vi "QR_code_Check_St2.vi"(5 "Columns":string[](array[string]), 8 "error in (no error)":errorcluster, 9 "replace %s":string, 10 "table":string, 11 "Refnum in":T1) -> (0 "error out":errorcluster, 2 "TRUE no barcode Done on station 1":bool, 3 "Refnum out":T1, 4 "FALSE healty":bool, 6 "resulting string":string, 7 "TRUE Duplication on Station 2":bool)   [LabVIEW 2017]
uses:
  <vilib>/addons/database/Connection.llb/Conn ObjectReference.ctl
  <vilib>/addons/database/NI_Database_API.lvlib
panel:
  out "data":string[][](array[string])
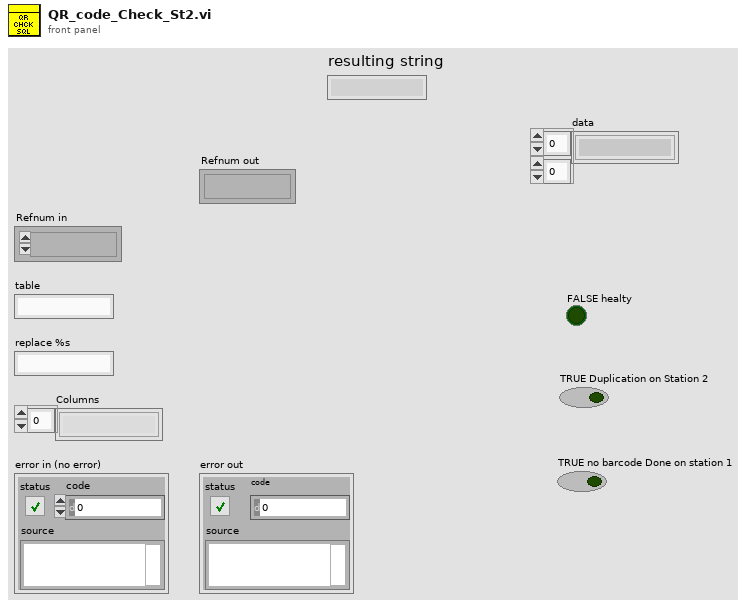
[diagram p1: front panel]
types:
  T1 = typedef "NI_Database_API.lvlib/Conn ObjectReference.ctl" = refnum<k1>
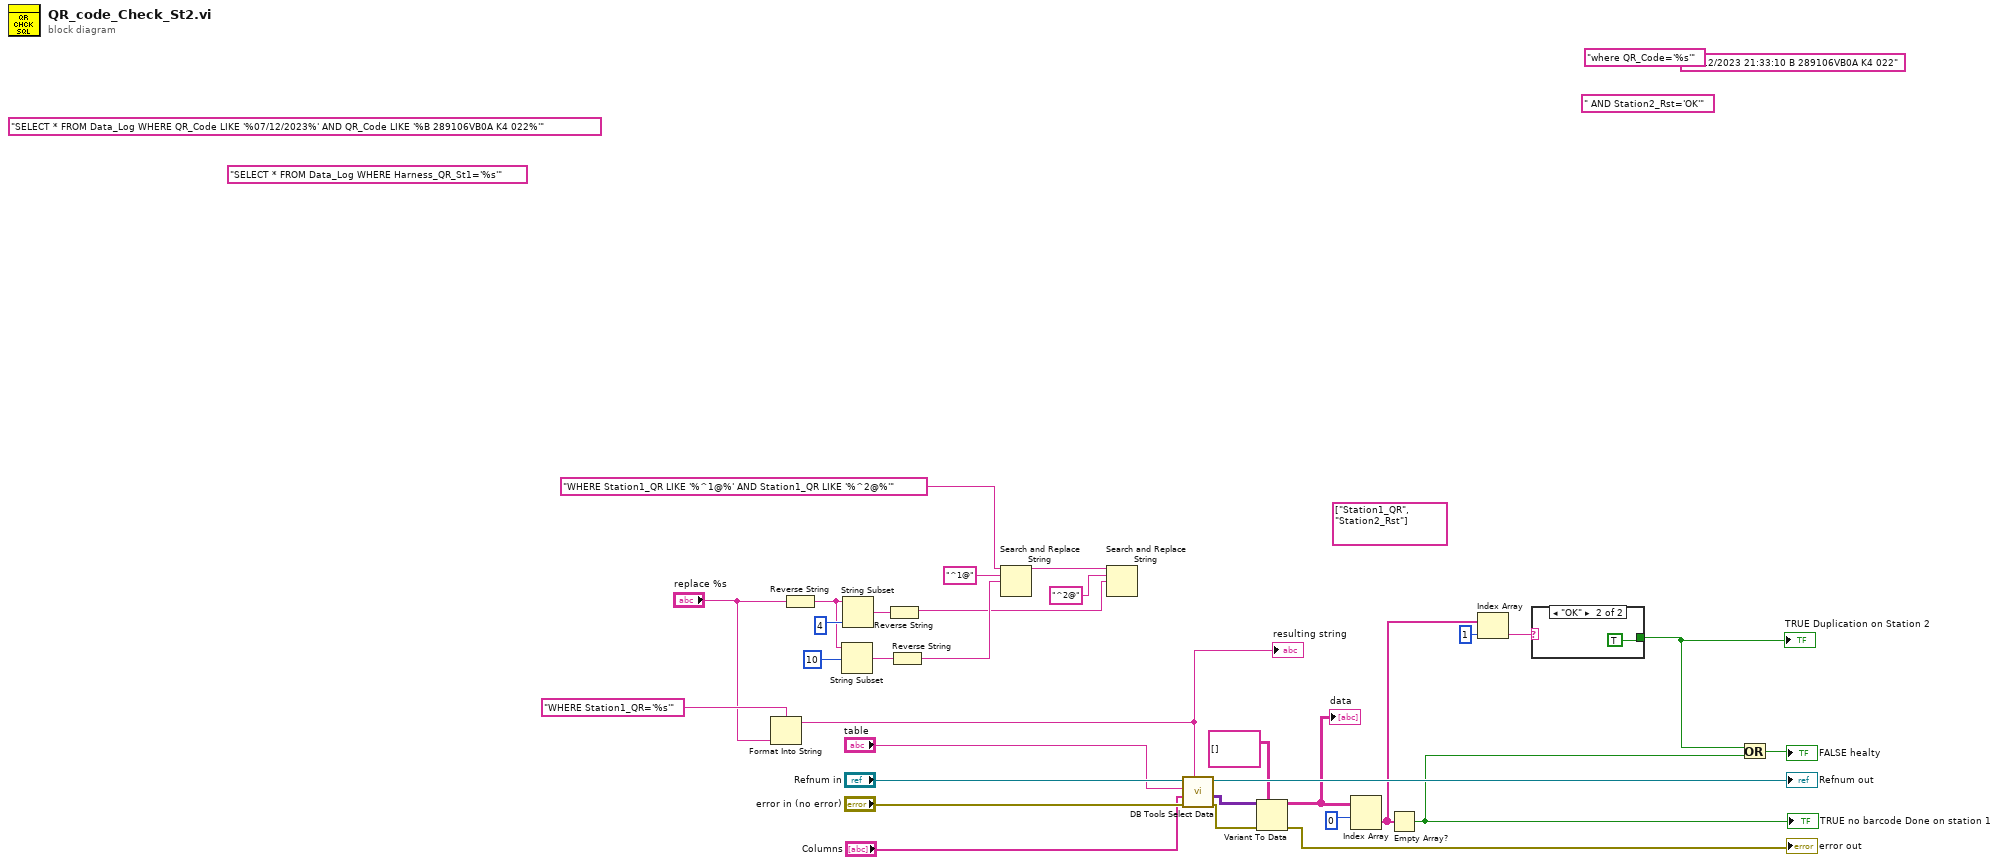
[diagram p0: block diagram]
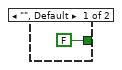
[diagram p2: hidden frame]
diagram:
  (unwired) string[] ["Station1_QR", "Station2_Rst"] ("columns 2")
  (unwired) "SELECT * FROM Data_Log WHERE Harness_QR_St1='%s'" ("format string")
  (unwired) "07/12/2023 21:33:10 B 289106VB0A K4 022" ("format string")
  (unwired) "SELECT * FROM Data_Log WHERE QR_Code LIKE '%07/12/2023%' AND QR_Code LIKE '%B 289106VB0A K4 022%'" ("format string")
  (unwired) "where QR_Code='%s'" ("format string")
  (unwired) " AND Station2_Rst='OK'" ("replace %s")
  n1 = Format Into String(format string="WHERE Station1_QR='%s'", "replace %s") -> (resulting string=w1:string)  [unwired: 2 in, 1 out]
  "resulting string" <- w1
  n2 = Reverse String(1:"replace %s") -> (0:w10:string)
  n3 = String Subset(string=w10, offset (0)=10) -> (substring=w9:string)  [unwired: 1 in]
  n4 = String Subset(string=w10, length (rest)=4 ("offset (0)")) -> (substring=w11:string)  [unwired: 1 in]
  n5 = Reverse String(1:w11) -> (0:w3:string)
  n6 = Reverse String(1:w9) -> (0:w4:string)
  n7 = Search and Replace String(input string="WHERE Station1_QR LIKE '%^1@%' AND Station1_QR LIKE '%^2@%'" ("format string"), search string="^1@", replace string=w4) -> (result string=w7:string)  [unwired: 5 in, 3 out]
  n8 = Search and Replace String(input string=w7, search string="^2@", replace string=w3) -> ()  [unwired: 5 in, 4 out]
  n9 = call <vilib>:"DB Tools Select Data.vi"("condition"=w1, "error in (no error)"="error in (no error)", "columns"="Columns", "table"="table", "connection reference"="Refnum in") -> ("error out"=w22:errorcluster, "data"=w24:variant[][], "connection reference out"=→"Refnum out":T1)  [unwired: 1 in]
  n10 = Variant To Data(error in=w22, type=string[][] [], Variant=w24) -> (data=w23:string[][], error out=→"error out":errorcluster)
  "data" <- w23
  n11 = Index Array(array=w23, index (row)=0) -> (element=w15:string[])  [unwired: 1 in]
  n12 = Empty Array?(array=w15) -> (empty?=w14:bool)
  "TRUE no barcode Done on station 1" <- w14
  n13 = Index Array(array=w15, index=1 ("index (row)")) -> (element=w18:string)
  n14 = case shown="\"OK\"" w18 {
    tunnel: [FALSE TRUE] -> w16
    frame "", Default {
    }
    frame "OK" {
    }
  }
  "TRUE Duplication on Station 2" <- w16
  n15 = Or(x=w16, y=w14) -> (x .or. y?=→"FALSE healty":bool)
